vi "Move.vi"(8 "Keypress In":enum16{"Right", "Down", "Up", "Left"}(ring), 9 "Map In":u32[][](array[numeric]), 10 "Locations In":cluster{"Location Y":i32, "Location X":i32}[](array[cluster])=[{"Location Y"=12, "Location X"=8}, {"Location Y"=12, "Location X"=7}, {"Location Y"=12, "Location X"=6}, {"Location Y"=12, "Location X"=5}, {"Location Y"=12, "Location X"=4}]) -> (1 "Keypress Out":enum16{"Right", "Down", "Up", "Left"}(ring), 2 "Map Out":u32[][](array[numeric]), 3 "Locations Out":cluster{"Location Y":i32, "Location X":i32}[](array[cluster]))   [LabVIEW 2014]
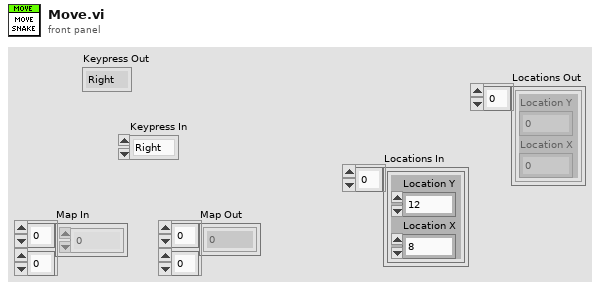
[diagram p1: front panel]
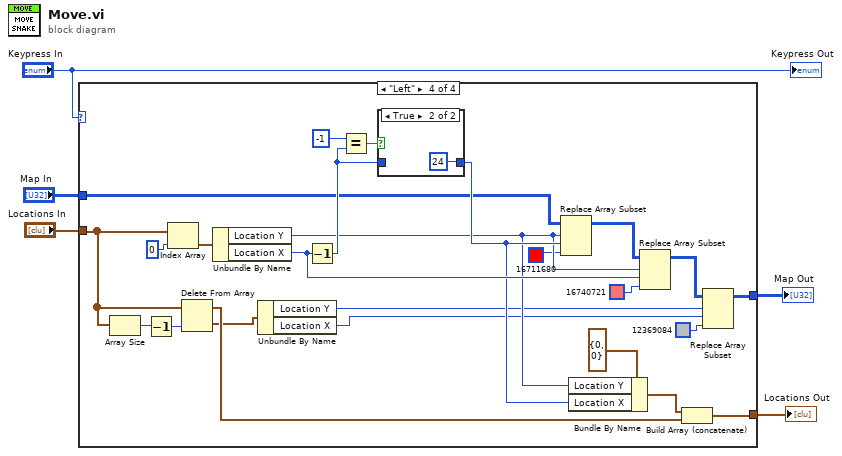
[diagram p0: block diagram]
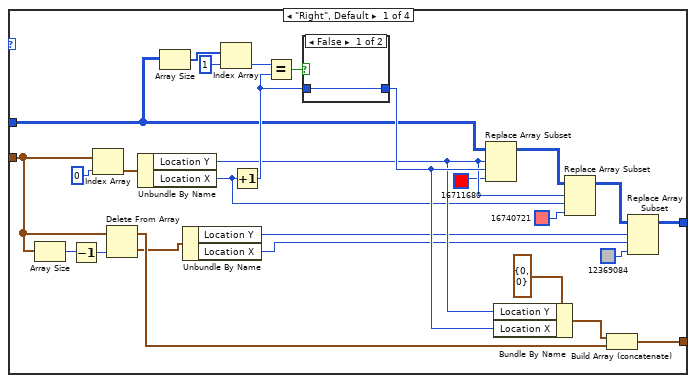
[diagram p2: hidden frame]
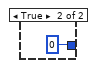
[diagram p3: hidden frame]
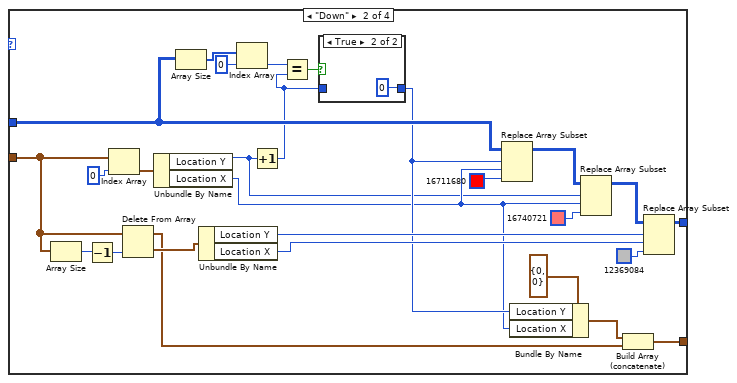
[diagram p4: hidden frame]
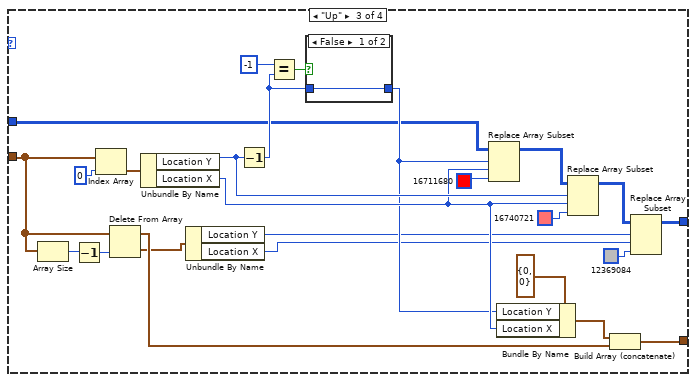
[diagram p6: hidden frame]
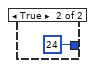
[diagram p7: hidden frame]
diagram:
  n1 = case shown="\"Left\"" "Keypress In" {
    tunnel: [w9 w55 w64 w91] -> w5
    tunnel: [w8 w48 w65 w92] -> w4
    tunnel: "Locations In" -> [w7 w47 w66 w93]
    tunnel: "Map In" -> [w6 w43 w67 w94]
    frame "Right", Default {
      n2 = Array Size(array=w7) -> (size(s)=w26:i32)
      n3 = Decrement(x=w26) -> (x-1=w25:i32)
      n4 = Index Array(array=w7, index=0) -> (element=w11:cluster{"Location Y":i32, "Location X":i32})
      n5 = Delete From Array(array=w7, index=w25) -> (deleted portion=w19:cluster{"Location Y":i32, "Location X":i32}, array with subset deleted=w21:cluster{"Location Y":i32, "Location X":i32}[])  [unwired: 1 in]
      n6 = Unbundle By Name(w11) -> ("Location Y"=w24:i32, "Location X"=w15:i32)
      n7 = Array Size(array=w6) -> (size(s)=w28:i32[])
      n8 = Unbundle By Name(w19) -> ("Location Y"=w18:i32, "Location X"=w20:i32)
      n9 = Index Array(array=w28, index=1) -> (element=w30:i32)
      n10 = Increment(x=w15) -> (x+1=w31:i32)
      n11 = Equal?(x=w30, y=w31) -> (x = y?=w27:bool)
      n12 = case shown="False" w27 {
        tunnel: w31 -> [w33 _]
        tunnel: [w33 0] -> w32
        frame False {
        }
        frame True {
        }
      }
      n13 = Replace Array Subset(array=w6, new element=u32 16711680, index (row)=w24, index (col)=w32) -> (w13:u32[][])
      n14 = Bundle By Name(cluster=cluster{"Location Y":i32, "Location X":i32} {"Location Y"=0, "Location X"=0} ("deleted portion"), "Location Y"=w24, "Location X"=w32) -> (w23:cluster{"Location Y":i32, "Location X":i32})
      n15 = Replace Array Subset(array=w13, new element=u32 16740721, index (row)=w24, index (col)=w15) -> (w16:u32[][])
      n16 = Build Array (concatenate)(w23, w21) -> (w8:cluster{"Location Y":i32, "Location X":i32}[])
      n17 = Replace Array Subset(array=w16, new element=u32 12369084, index (row)=w18, index (col)=w20) -> (w9:u32[][])
    }
    frame "Down" {
      n18 = Array Size(array=w47) -> (size(s)=w45:i32)
      n19 = Decrement(x=w45) -> (x-1=w46:i32)
      n20 = Index Array(array=w47, index=0) -> (element=w60:cluster{"Location Y":i32, "Location X":i32})
      n21 = Delete From Array(array=w47, index=w46) -> (deleted portion=w53:cluster{"Location Y":i32, "Location X":i32}, array with subset deleted=w51:cluster{"Location Y":i32, "Location X":i32}[])  [unwired: 1 in]
      n22 = Unbundle By Name(w60) -> ("Location Y"=w35:i32, "Location X"=w37:i32)
      n23 = Array Size(array=w43) -> (size(s)=w42:i32[])
      n24 = Unbundle By Name(w53) -> ("Location Y"=w54:i32, "Location X"=w52:i32)
      n25 = Index Array(array=w42, index=0) -> (element=w40:i32)
      n26 = Increment(x=w35) -> (x+1=w39:i32)
      n27 = Equal?(x=w40, y=w39) -> (x = y?=w44:bool)
      n28 = case shown="True" w44 {
        tunnel: w39 -> [w62 _]
        tunnel: [w62 0] -> w38
        frame False {
        }
        frame True {
        }
      }
      n29 = Replace Array Subset(array=w43, new element=u32 16711680, index (row)=w38, index (col)=w37) -> (w59:u32[][])
      n30 = Bundle By Name(cluster=cluster{"Location Y":i32, "Location X":i32} {"Location Y"=0, "Location X"=0} ("deleted portion"), "Location Y"=w38, "Location X"=w37) -> (w49:cluster{"Location Y":i32, "Location X":i32})
      n31 = Replace Array Subset(array=w59, new element=u32 16740721, index (row)=w35, index (col)=w37) -> (w57:u32[][])
      n32 = Build Array (concatenate)(w49, w51) -> (w48:cluster{"Location Y":i32, "Location X":i32}[])
      n33 = Replace Array Subset(array=w57, new element=u32 12369084, index (row)=w54, index (col)=w52) -> (w55:u32[][])
    }
    frame "Up" {
      n34 = Array Size(array=w66) -> (size(s)=w81:i32)
      n35 = Decrement(x=w81) -> (x-1=w80:i32)
      n36 = Index Array(array=w66, index=0) -> (element=w69:cluster{"Location Y":i32, "Location X":i32})
      n37 = Delete From Array(array=w66, index=w80) -> (deleted portion=w75:cluster{"Location Y":i32, "Location X":i32}, array with subset deleted=w77:cluster{"Location Y":i32, "Location X":i32}[])  [unwired: 1 in]
      n38 = Unbundle By Name(w69) -> ("Location Y"=w86:i32, "Location X"=w84:i32)
      n39 = Unbundle By Name(w75) -> ("Location Y"=w74:i32, "Location X"=w76:i32)
      n40 = Decrement(x=w86) -> (x-1=w87:i32)
      n41 = Equal?(x=-1, y=w87) -> (x = y?=w82:bool)
      n42 = case shown="False" w82 {
        tunnel: w87 -> [w89 _]
        tunnel: [w89 24] -> w83
        frame False {
        }
        frame True {
        }
      }
      n43 = Replace Array Subset(array=w67, new element=u32 16711680, index (row)=w83, index (col)=w84) -> (w70:u32[][])
      n44 = Bundle By Name(cluster=cluster{"Location Y":i32, "Location X":i32} {"Location Y"=0, "Location X"=0} ("deleted portion"), "Location Y"=w83, "Location X"=w84) -> (w79:cluster{"Location Y":i32, "Location X":i32})
      n45 = Replace Array Subset(array=w70, new element=u32 16740721, index (row)=w86, index (col)=w84) -> (w72:u32[][])
      n46 = Build Array (concatenate)(w79, w77) -> (w65:cluster{"Location Y":i32, "Location X":i32}[])
      n47 = Replace Array Subset(array=w72, new element=u32 12369084, index (row)=w74, index (col)=w76) -> (w64:u32[][])
    }
    frame "Left" {
      n48 = Array Size(array=w93) -> (size(s)=w110:i32)
      n49 = Decrement(x=w110) -> (x-1=w109:i32)
      n50 = Index Array(array=w93, index=0) -> (element=w96:cluster{"Location Y":i32, "Location X":i32})
      n51 = Delete From Array(array=w93, index=w109) -> (deleted portion=w103:cluster{"Location Y":i32, "Location X":i32}, array with subset deleted=w105:cluster{"Location Y":i32, "Location X":i32}[])  [unwired: 1 in]
      n52 = Unbundle By Name(w96) -> ("Location Y"=w108:i32, "Location X"=w113:i32)
      n53 = Unbundle By Name(w103) -> ("Location Y"=w102:i32, "Location X"=w104:i32)
      n54 = Decrement(x=w113) -> (x-1=w114:i32)
      n55 = Equal?(x=-1, y=w114) -> (x = y?=w111:bool)
      n56 = case shown="True" w111 {
        tunnel: w114 -> [w116 _]
        tunnel: [w116 24] -> w112
        frame False {
        }
        frame True {
        }
      }
      n57 = Replace Array Subset(array=w94, new element=u32 16711680, index (row)=w108, index (col)=w112) -> (w98:u32[][])
      n58 = Bundle By Name(cluster=cluster{"Location Y":i32, "Location X":i32} {"Location Y"=0, "Location X"=0} ("deleted portion"), "Location Y"=w108, "Location X"=w112) -> (w107:cluster{"Location Y":i32, "Location X":i32})
      n59 = Replace Array Subset(array=w98, new element=u32 16740721, index (row)=w108, index (col)=w113) -> (w100:u32[][])
      n60 = Build Array (concatenate)(w107, w105) -> (w92:cluster{"Location Y":i32, "Location X":i32}[])
      n61 = Replace Array Subset(array=w100, new element=u32 12369084, index (row)=w102, index (col)=w104) -> (w91:u32[][])
    }
  }
  "Map Out" <- w5
  "Locations Out" <- w4
  "Keypress Out" <- "Keypress In"
